vi "fire error object.vi"(10 "Error in":refnum<class>, 11 "Template in":refnum<class "Template.lvclass">) -> ()   [LabVIEW 2020, in "Template.lvlib" / "Template.lvclass"]
uses:
  Template.lvclass
  Template.lvclass/Template.ctl
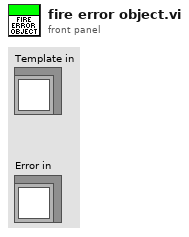
[diagram p1: front panel]
types:
  T1 = typedef "Template.lvlib/Template.lvclass/base actor events.ctl" = cluster{"Stop Actor":refnum<user-event>, "New Error":refnum<user-event>, "New Settings":refnum<user-event>}
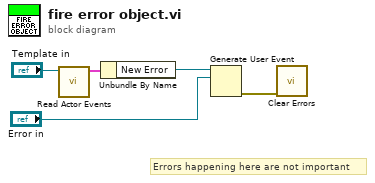
[diagram p0: block diagram]
diagram:
  # "Errors happening here are not important"
  n1 = call "Read Actor Events.vi"("Template in"="Template in") -> ("Base Actor Events"=w3:T1)  [unwired: 10 in]
  n2 = Unbundle By Name(w3) -> ("New Error"=w5:refnum<user-event>)
  n3 = Generate User Event(user event=w5, event data cluster="Error in") -> (error out=w2:errorcluster)  [unwired: 2 in, 1 out]
  n4 = call <vilib>:"Clear Errors.vi"("error in (no error)"=w2) -> ()  [unwired: 5 in, 2 out]
